vi "streamToDisk.vi"(8 "error in (no error)":errorcluster, 9 "sampleRate":i32=96000, 10 "singleToneData":T1(array[cluster]), 11 "SoundDeviceData in":refnum<class "SoundDeviceData.lvclass">) -> (0 "error out":errorcluster, 1 "times":dbl[](array[numeric]), 2 "Path":path, 3 "SoundDeviceData out":refnum<class "SoundDeviceData.lvclass">)   [LabVIEW 2011, in "DataMappers.lvlib" / "SoundDeviceData.lvclass"]
uses:
  SoundDeviceData.lvclass
  DatabaseHelpers/Database Objects/Channel/Channel.lvclass
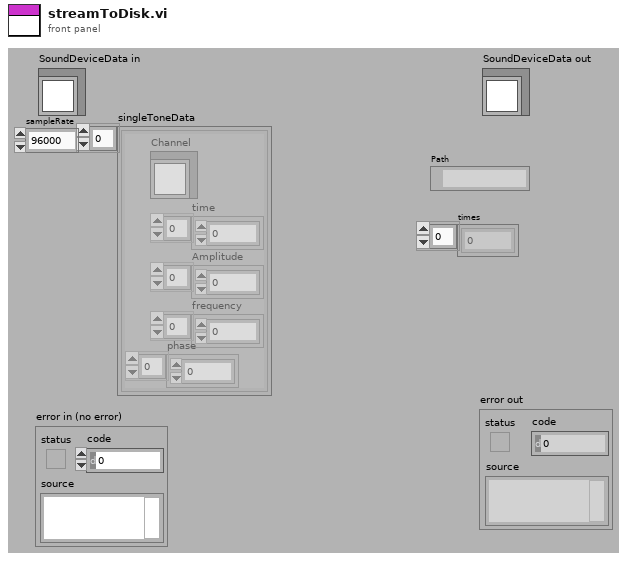
[diagram p1: front panel]
types:
  T1 = cluster{"Channel":refnum<class "Channel.lvclass">, "time":dbl[], "Amplitude":dbl[], "frequency":dbl[], "phase":dbl[]}[]
  T2 = cluster{"Channel":refnum<class "Channel.lvclass">, "time":dbl[], "Amplitude":dbl[], "frequency":dbl[], "phase":dbl[]}
  T3 = cluster{"Channel":refnum<class "Channel.lvclass">, "sampleSegements":dbl[], "Amplitude":dbl[], "frequency":dbl[], "phase":dbl[]}[]
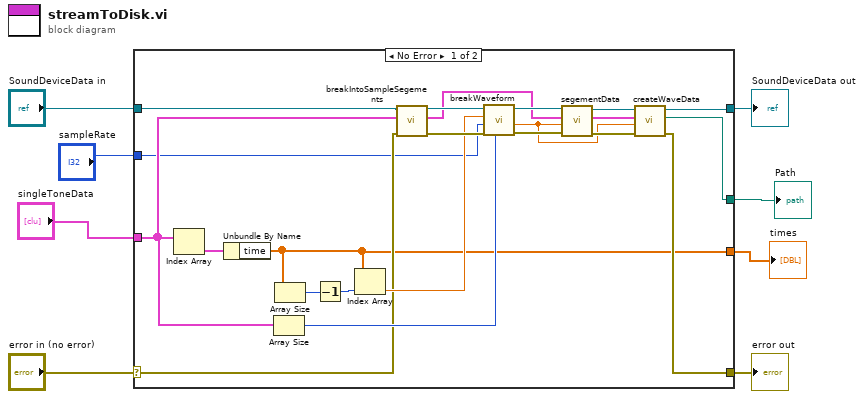
[diagram p0: block diagram]
diagram:
  n1 = case shown="No Error" "error in (no error)" {
    selector: "error in (no error)" -> [w13 w32]
    tunnel: [w12 w32] -> w7
    tunnel: [w15 w31] -> w5
    tunnel: "SoundDeviceData in" -> [w16 w31]
    tunnel: "singleToneData" -> [w14 _]
    tunnel: [w11 _] -> w3
    tunnel: [w10 _] -> w2
    tunnel: "sampleRate" -> [w9 _]
    frame No Error {
      n2 = Index Array(array=w14) -> (element=w26:T2)  [unwired: 1 in]
      n3 = Unbundle By Name(w26) -> ("time"=w10:dbl[])
      n4 = Array Size(array=w14) -> (size(s)=w22:i32)
      n5 = Array Size(array=w10) -> (size(s)=w25:i32)
      n6 = Decrement(x=w25) -> (x-1=w24:i32)
      n7 = Index Array(array=w10, index=w24) -> (element=w23:dbl)
      n8 = call "breakIntoSampleSegements.vi"("error in (no error)"=w13, "singleToneData"=w14, "SoundDeviceData in"=w16) -> ("error out"=w27:errorcluster, "segmentedData"=w28:T3, "SoundDeviceData out"=w29:refnum<class "SoundDeviceData.lvclass">)  [unwired: 6 in]
      n9 = call "breakWaveform.vi"("ChannelNumber"=w22, "error in (no error)"=w27, "samplingRate"=w9, "total duration"=w23, "SoundDeviceData in"=w29) -> ("error out"=w20:errorcluster, "samplePerChunkPerChannel"=w17:dbl, "SoundDeviceData out"=w30:refnum<class "SoundDeviceData.lvclass">)  [unwired: 3 in, 1 out]
      n10 = call "segementData.vi"("error in (no error)"=w20, "samplesPerChunkPerChannel"=w17, "segmentedData"=w28, "SoundDeviceData in"=w30) -> ("error out"=w19:errorcluster, "segementData"=w21:T3, "SoundDeviceData out"=w18:refnum<class "SoundDeviceData.lvclass">)  [unwired: 5 in]
      n11 = call "createWaveData.vi"("error in (no error)"=w19, "samplesPerChunkPerChannel"=w17, "segementData"=w21, "SoundDeviceData in"=w18) -> ("error out"=w12:errorcluster, "Path"=w11:path, "SoundDeviceData out"=w15:refnum<class "SoundDeviceData.lvclass">)  [unwired: 5 in]
    }
    frame Error {
    }
  }
  "error out" <- w7
  "SoundDeviceData out" <- w5
  "Path" <- w3
  "times" <- w2
